vi "SetTriggerEnabled.vi"(8 "error in":errorcluster, 10 "trigger":bool=TRUE, 11 "camera.nit in":refnum<class "camera.lvclass">) -> (0 "error out":errorcluster)   [LabVIEW 2020, in "camera.lvclass"]
uses:
  camera.lvclass
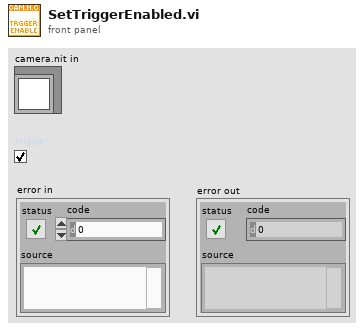
[diagram p1: front panel]
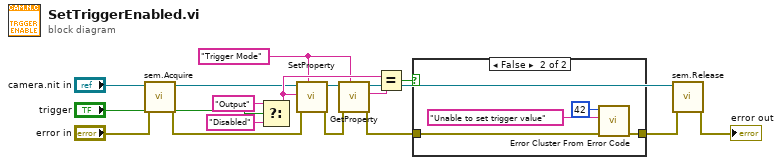
[diagram p0: block diagram]
diagram:
  w8 = "Trigger Mode" ("pPrp")
  n1 = call "sem.Acquire.vi"("error in"="error in", "camera.nit in"="camera.nit in") -> ("error out"=w4:errorcluster)  [unwired: 9 in]
  n2 = Select(t="Output" ("Value"), s="trigger", f="Disabled") -> (s? t:f=w12:string)
  n3 = call-dynamic "SetProperty.vi"("Property"=w8, "error in"=w4, "Value"=w12, "camera.nit in"="camera.nit in") -> ("error out"=w7:errorcluster)  [unwired: 7 in]
  n4 = call-dynamic "GetProperty.vi"("Property"=w8, "error in"=w7, "camera.nit in"="camera.nit in") -> ("error out"=w9:errorcluster, "value"=w13:string)  [unwired: 7 in]
  n5 = Equal?(x=w12, y=w13) -> (x = y?=w14:bool)
  n6 = case shown="False" w14 {
    tunnel: w9 -> [w15 w19]
    tunnel: [w15 w17] -> w2
    frame True {
    }
    frame False {
      n7 = call <vilib>:"Error Cluster From Error Code.vi"("error in (no error)"=w19, "error message (\"\")"="Unable to set trigger value" ("error message (\"\")"), "error code (0)"=42) -> ("error out"=w17:errorcluster)  [unwired: 6 in]
    }
  }
  n8 = call "sem.Release.vi"("error in"=w2, "camera.nit in"="camera.nit in") -> ("error out"=→"error out":errorcluster)  [unwired: 9 in]
